vi "Motor conditions_subVI.vi"(0 "Target Angle (°)":dbl, 5 "Pot. Read (V)":dbl, 9 "Stop":bool, 11 "error in (no error)":errorcluster) -> (4 "Motor On/Off":bool, 6 "Motor FWD/RVS":bool, 15 "error out":errorcluster)   [LabVIEW 2017]
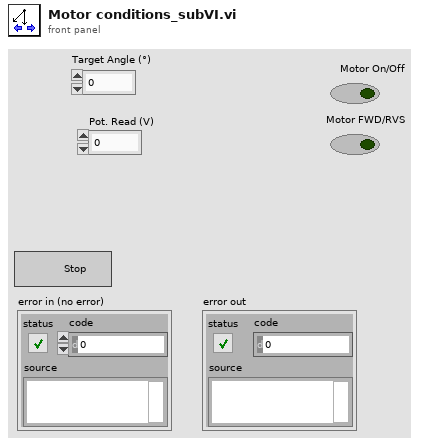
[diagram p1: front panel]
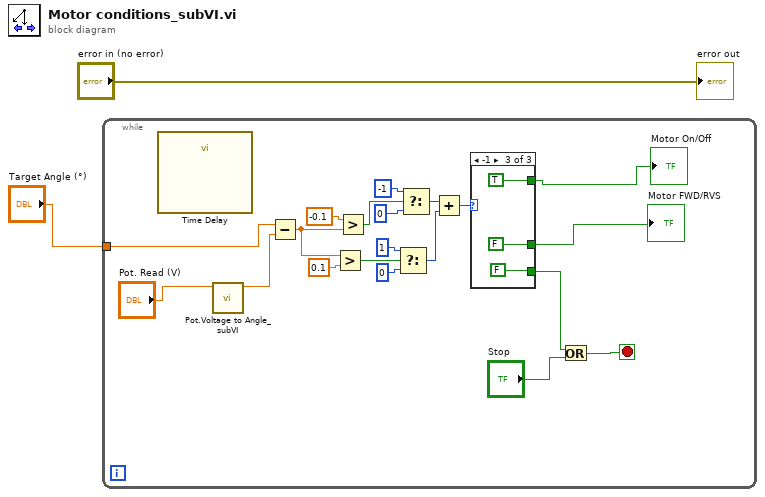
[diagram p0: block diagram]
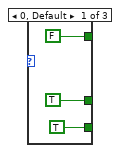
[diagram p2: hidden frame]
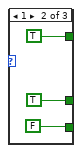
[diagram p3: hidden frame]
diagram:
  n1 = while {
    tunnel: "Target Angle (°)" -> [w8]
    stop <- w10 stop-if-true
    n2 = call "Time Delay"() -> ()  [unwired: 11 in, 1 out]
    n3 = call "Pot.Voltage to Angle_subVI.vi"("Potentiometer V (0-5)"="Pot. Read (V)") -> ("Pull-back angle (°)"=w3:dbl)  [unwired: 10 in]
    n4 = Subtract(x=w8, y=w3) -> (x-y=w21:dbl)
    n5 = Greater?(x=w21, y=0.1) -> (0:w16:bool)
    n6 = Greater?(x=-0.1, y=w21) -> (0:w19:bool)
    n7 = Select(t=1, s=w16, f=0) -> (s? t:f=w12:i32)
    n8 = Select(t=-1, s=w19, f=0) -> (s? t:f=w13:i32)
    n9 = Add(x=w13, y=w12) -> (x+y=w11:i32)
    n10 = case shown="-1" w11 {
      tunnel: [TRUE TRUE FALSE] -> w6
      tunnel: [FALSE TRUE TRUE] -> w7
      tunnel: [TRUE FALSE FALSE] -> w9
      frame 0, Default {
      }
      frame 1 {
      }
      frame -1 {
      }
    }
    "Motor FWD/RVS" <- w6
    "Motor On/Off" <- w7
    n11 = Or(x=w9, y="Stop") -> (x .or. y?=w10:bool)
  }
  "error out" <- "error in (no error)"
